vi "Center Object.vi"(8 "error in":errorcluster, 9 "Rectangle":T1, 10 "Scrollbar Visible?":bool, 11 "SubPanel in":refnum<class "SubPanel.lvclass">) -> (0 "error out":errorcluster, 3 "SubPanel out":refnum<class "SubPanel.lvclass">)   [LabVIEW 2012, in "SubPanel.lvlib" / "SubPanel.lvclass"]
uses:
  SubPanel.lvclass
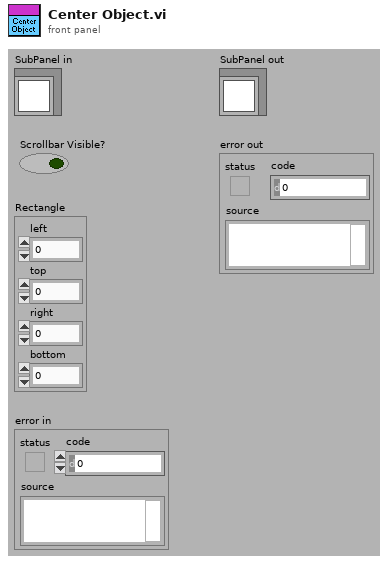
[diagram p1: front panel]
types:
  T1 = cluster{"left":i16, "top":i16, "right":i16, "bottom":i16}
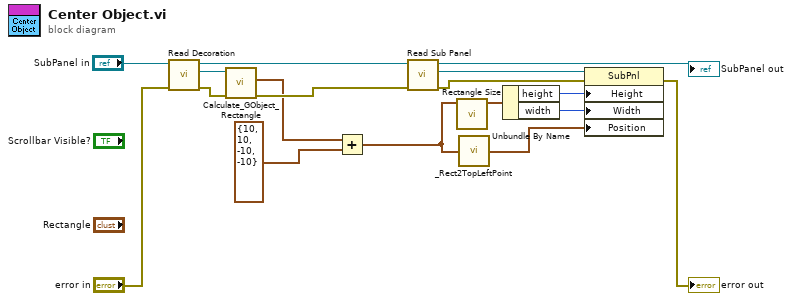
[diagram p0: block diagram]
diagram:
  n1 = call-dynamic "Read Decoration.vi"("error in (no error)"="error in", "Dialog.lvclass in"="SubPanel in") -> ("error out"=w5:errorcluster, "Decoration"=w6:refnum<vi>, "Dialog.lvclass out"=w8:refnum<class "SubPanel.lvclass">)  [unwired: 7 out]
  n2 = call "Calculate_GObject_Rectangle.vi"("error in"=w5, "GObject ref"=w6) -> ("error out"=w4:errorcluster, "Rectangle"=w3:T1)  [unwired: 8 out]
  n3 = Add(x=w3, y=T1 {"left"=10, "top"=10, "right"=-10, "bottom"=-10}) -> (x+y=w1:T1)
  n4 = call-dynamic "Read Sub Panel.vi"("error in (no error)"=w4, "SubPanel.lvclass in"=w8) -> ("error out"=w11:errorcluster, "Sub Panel"=w12:refnum<vi>, "SubPanel.lvclass out"=→"SubPanel out":refnum<class "SubPanel.lvclass">)  [unwired: 7 out]
  n5 = call "Rectangle Size.vi"("Rectangle"=w1) -> ("Rect Size"=w16:cluster{"width":i32, "height":i32})  [unwired: 10 out]
  n6 = call "_Rect2TopLeftPoint.vi"("bounds"=w1) -> ("TopLeft point"=w17:cluster{"x":i32, "y":i32})  [unwired: 4 out]
  n7 = Unbundle By Name(w16) -> ("height"=w14:i32, "width"=w15:i32)
  n8 = property class="SubPnl"(reference=w12, error in=w11, "Height"=w14, "Width"=w15, "Position"=w17) -> (error out=→"error out":errorcluster)  [unwired: 1 out]
